vi "Read RFFE Waveform.vi"(7 "Number of Registers to Read":u8, 8 "error in (no error)":errorcluster, 9 "Reg_Address_Data":T1={"Address"=81, "Data"=0} {"Address" format="%.0x"}, 10 "USID":T2 max=15, 11 "HSDIO_VISA":refnum<k15> caption="HSDIO_Acq_Visa") -> (0 "error out":errorcluster, 1 "Waveform Graph":digitalwaveform(graph), 2 "Ext_Read_Data":u8[](array[numeric])=[31, 144, 7], 3 "Ext_Read_Reg":i32[](array[numeric]), 4 "Converted Data":T3 {"Register" max=31 format="%.0x"; "Slave Address" max=15 format="%.0x"})   [LabVIEW 2013]
uses:
  Controls/USID.ctl
  Controls/Reg_Address_Data.ctl
  Instruments/HSDIO/MIPI_RFFE/Ctrls/Configuration.ctl
  Instruments/HSDIO/MIPI_RFFE/Ctrls/ClockDataChannels.ctl
  Instruments/HSDIO/MIPI_RFFE/Ctrls/RegReadWrite.ctl
  <vilib>/Waveform/DWDTOps.llb/DWDT Digital Size.vi
  <instrlib>/niHSDIO/niHSDIO.llb/niHSDIO Write Named Waveform (WDT).vi
  <instrlib>/niHSDIO/niHSDIO.llb/niHSDIO Fetch Waveform (WDT).vi
panel:
  in  "Specific Bits Value_to_Read":cluster{"#ofBits":u8, "Bit_Location(LSB)":u8}={"#ofBits"=1, "Bit_Location(LSB)"=0} {"Bit_Location(LSB)" max=7; "#ofBits" min=1 max=8}
  out "Specific_Bits_Value":u8=184
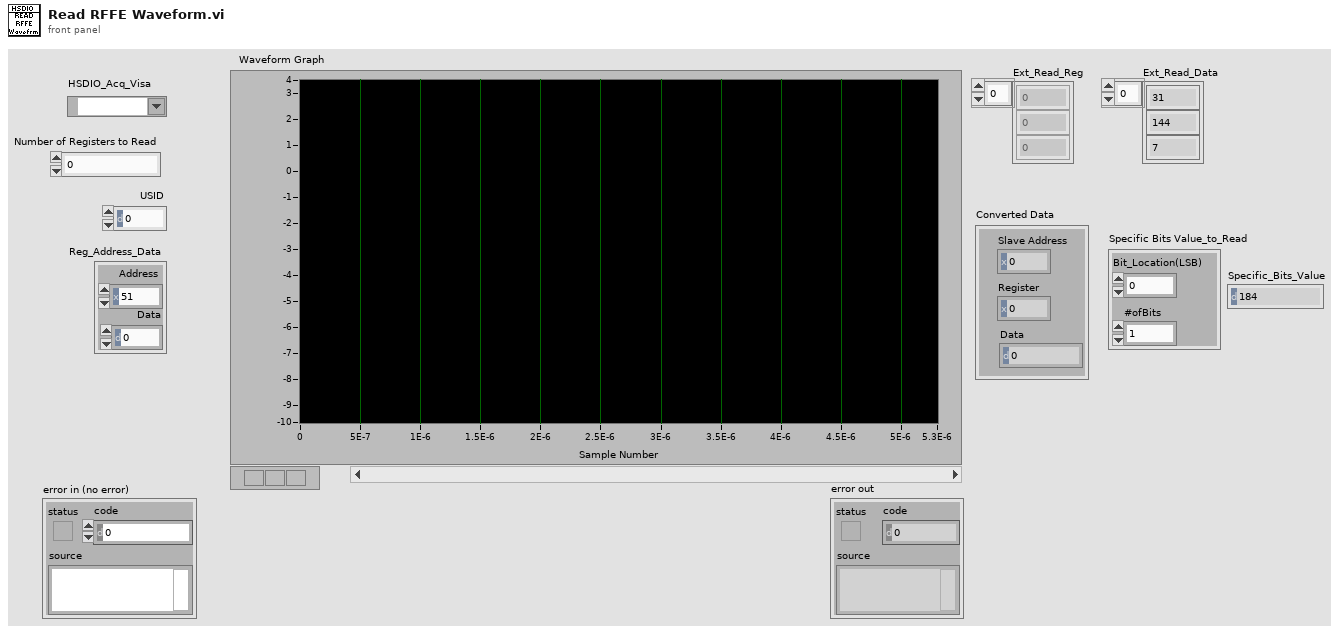
[diagram p1: front panel]
types:
  T1 = typedef "Reg_Address_Data.ctl" = cluster{"Address":u8, "Data":u8}
  T2 = typedef "USID.ctl" = u8
  T3 = cluster{"Slave Address":u8, "Register":u8, "Data":u8}
  T4 = typedef "RegReadWrite.ctl" = cluster{"Slave Address":u8, "Register":u8, "Data":u8, "SetID_Pin_State":enum16{"0", "1", "Z"}}
  T5 = typedef "Configuration.ctl" = cluster{"Samples to Allocate":i32, "Oversample Factor":u8, "Clock Channel":T6, "Data Channel":T6}
  T6 = typedef "ClockDataChannels.ctl" = enum16{"0", "1"}
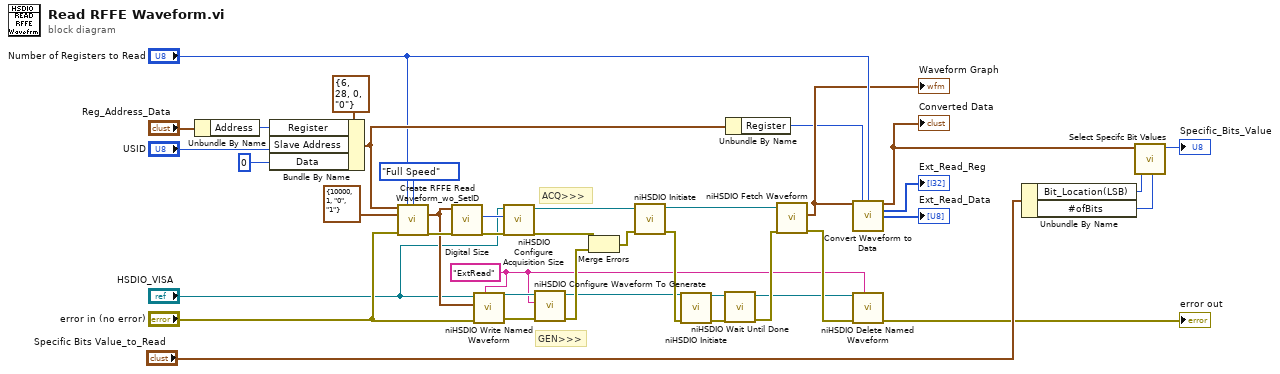
[diagram p0: block diagram]
diagram:
  w15 = "ExtRead" ("waveform name (default:\"\")")
  # "GEN>>>"
  # "ACQ>>>"
  n1 = Unbundle By Name("Reg_Address_Data") -> ("Address"=w1:u8)
  n2 = Bundle By Name(cluster=T4 {"Slave Address"=6, "Register"=28, "Data"=0, "SetID_Pin_State"=enum."0"} ("Data"), "Register"=w1, "Slave Address"="USID", "Data"=u8 0) -> (w37:T4)
  n3 = call "Create RFFE Read Waveform_wo_SetID.vi"("Data"=w37, "Ext_Read_Num_Reg"="Number of Registers to Read", "Readback Speed"=enum16{"Full Speed", "Half Speed"}."Full Speed", "Configuratation"=T5 {"Samples to Allocate"=10000, "Oversample Factor"=1, "Clock Channel"=enum."0", "Data Channel"=enum."1"}, "error in (no error)"="error in (no error)") -> ("Waveform Graph"=w13:digitalwaveform, "error out"=w27:errorcluster)  [unwired: 9 in]
  n4 = call-poly <vilib>:"Digital Size.vi"("error in (no error)"=w27, "digital waveform in"=w13) -> ("error out"=w28:errorcluster, "number of samples"=w29:i32)  [unwired: 6 in, 2 out]
  n5 = call-poly <instrlib>:"niHSDIO Write Named Waveform.vi"("waveform name (default:\"\")"=w15, "error in (no error)"="error in (no error)", "data"=w13, "instrument handle"="HSDIO_VISA") -> ("error out"=w21:errorcluster, "instrument handle out"=w19:refnum<k15>)  [unwired: 6 in]
  n6 = call <instrlib>:"niHSDIO Configure Acquisition Size.vi"("error in (no error)"=w28, "samples per record (1000 samples)"=w29, "instrument handle"="HSDIO_VISA") -> ("error out"=w26:errorcluster, "instrument handle out"=w30:refnum<k15>)  [unwired: 7 in]
  n7 = call <instrlib>:"niHSDIO Configure Waveform To Generate.vi"("error in (no error)"=w21, "waveform name"=w15, "instrument handle"=w19) -> ("error out"=w20:errorcluster, "instrument handle out"=w18:refnum<k15>)  [unwired: 7 in]
  n8 = Merge Errors(w26, w20) -> (w31:errorcluster)
  n9 = call <instrlib>:"niHSDIO Initiate.vi"("error in (no error)"=w31, "instrument handle"=w30) -> ("error out"=w33:errorcluster, "instrument handle out"=w22:refnum<k15>)  [unwired: 8 in]
  n10 = call <instrlib>:"niHSDIO Initiate.vi"("error in (no error)"=w33, "instrument handle"=w18) -> ("error out"=w32:errorcluster, "instrument handle out"=w23:refnum<k15>)  [unwired: 8 in]
  n11 = call <instrlib>:"niHSDIO Wait Until Done.vi"("error in (no error)"=w32, "instrument handle"=w23) -> ("error out"=w25:errorcluster, "instrument handle out"=w16:refnum<k15>)  [unwired: 8 in]
  n12 = Unbundle By Name(w37) -> ("Register"=w10:u8)
  n13 = call-poly <instrlib>:"niHSDIO Fetch Waveform.vi"("error in (no error)"=w25, "instrument handle"=w22) -> ("error out"=w17:errorcluster, "data"=w14:digitalwaveform)  [unwired: 6 in, 2 out]
  "Waveform Graph" <- w14
  n14 = call "Convert Waveform to Data.vi"("Waveform Graph"=w14, "Register"=w10, "Ext_Read_Num_Reg"="Number of Registers to Read") -> ("Converted Data"=w9:T3, "Ext_Read_Reg"=→"Ext_Read_Reg":i32[], "Ext_Read_Data"=→"Ext_Read_Data":u8[])  [unwired: 10 in]
  "Converted Data" <- w9
  n15 = call <instrlib>:"niHSDIO Delete Named Waveform.vi"("waveform name (default:\"\")"=w15, "error in (no error)"=w17, "instrument handle"=w16) -> ("error out"=→"error out":errorcluster)  [unwired: 7 in, 1 out]
  n16 = Unbundle By Name("Specific Bits Value_to_Read") -> ("Bit_Location(LSB)"=w8:u8, "#ofBits"=w7:u8)
  n17 = call "Select Specifc Bit Values.vi"("#ofBits"=w7, "Bit_Location(LSB)"=w8, "Converted Data"=w9) -> ("Bits"=→"Specific_Bits_Value":u8)  [unwired: 8 in]
